vi "Main.vi"() -> ()   [LabVIEW 2015]
doc: "This software acquires data from a simulated source, displays it and performs analysis of the data."
uses:
  Controls/State.ctl
  Controls/Data.ctl
  Controls/Configuration Settings.ctl
  Controls/File Type.ctl
panel:
  in  "File Type":T1
  in  "Open File Location":bool
  in  "Open":bool
  in  "Save":bool
  out "Current State":string
  out "Data":dbl[](graph)
  in  "Reset Settings":bool
  in  "Clear Graph":bool
  in  "Analyze Data":bool
  in  "Acquire Data":bool
  in  "Configure Data":bool
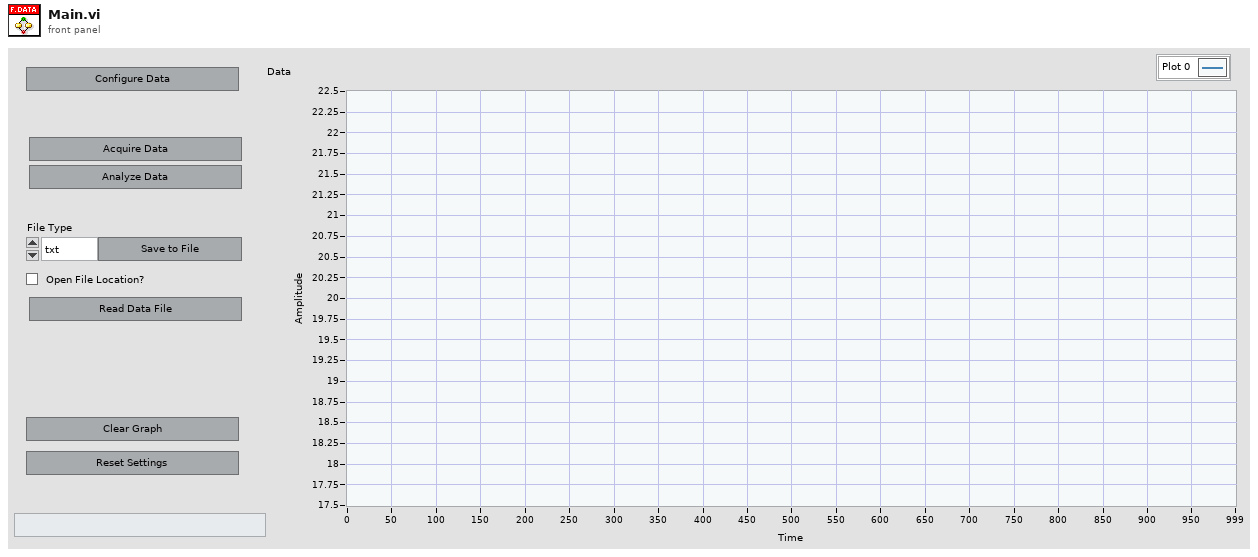
[diagram p1: front panel]
types:
  T1 = typedef "File Type.ctl" = enum16{"txt", "csv", "tdms"}
  T2 = typedef "Data.ctl" = cluster{"Configuration Settings":T3, "Data":dbl[]}
  T3 = typedef "Configuration Settings.ctl" = cluster{"Offset":dbl, "Signal Type":enum16{"Sine Wave", "Triangle Wave", "Square Wave", "Sawtooth Wave"}, "Frequency":dbl, "Amplitude":dbl, "Phase":dbl, "Noise Amplitude":dbl}
  T4 = typedef "State.ctl" = enum16{"Initialize", "Wait for Event", "Configure", "Acquire Data", "Update User Interface", "Reset Data", "Open Data File", "Save Data File", "Clear Data", "Analyse Data", "Stop", "Error"}
  T5 = enum16{"Sine Wave", "Triangle Wave", "Square Wave", "Sawtooth Wave"}
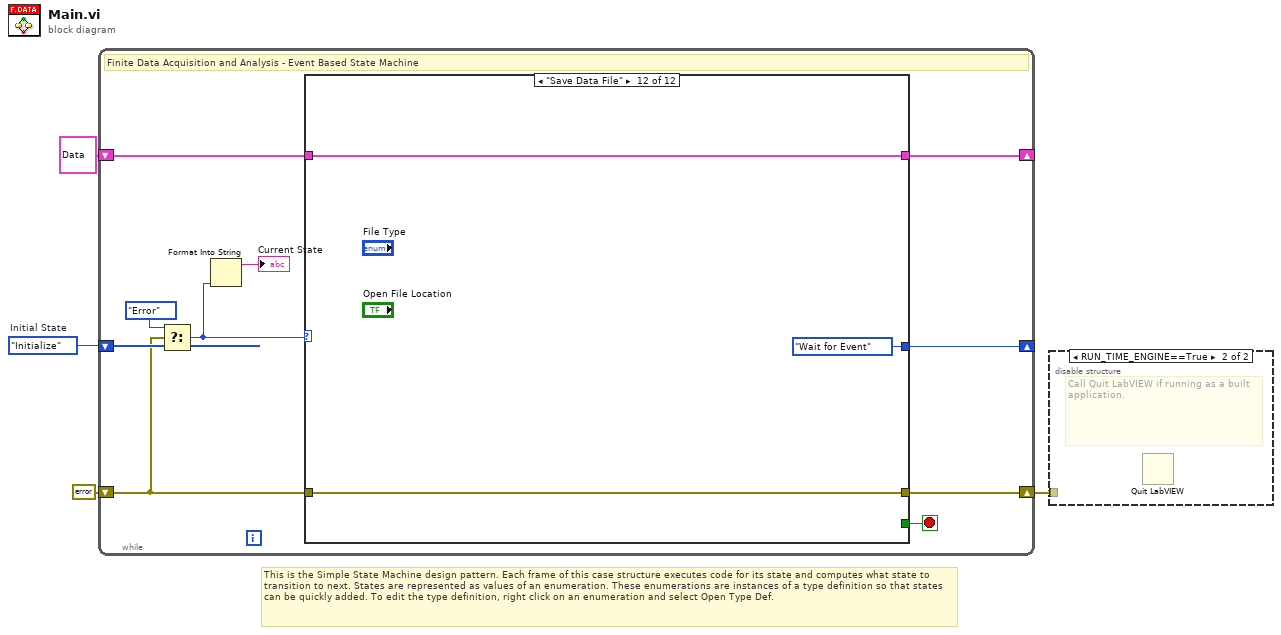
[diagram p0: block diagram]
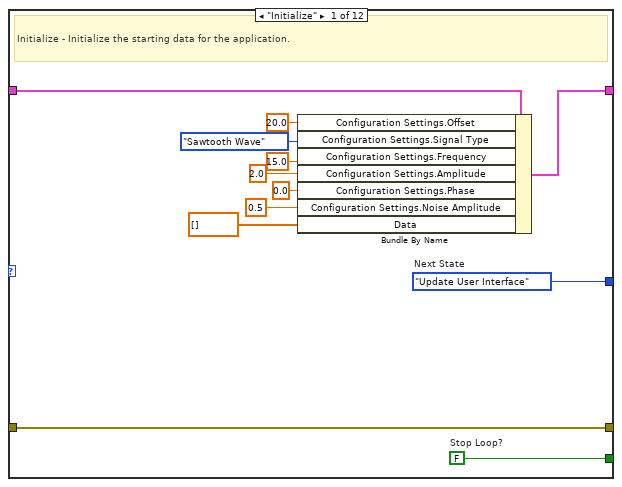
[diagram p2: hidden frame]
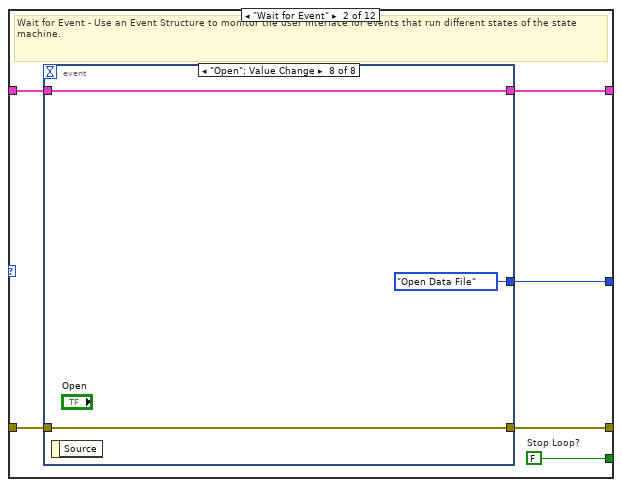
[diagram p3: hidden frame]
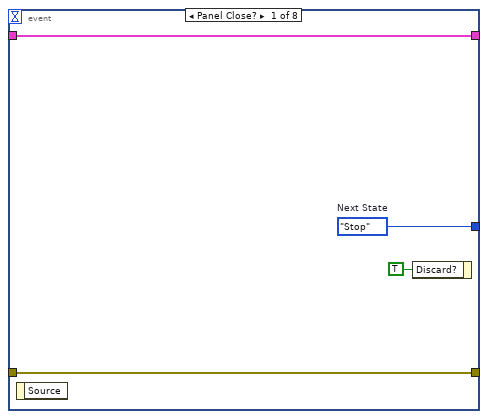
[diagram p4: hidden frame]
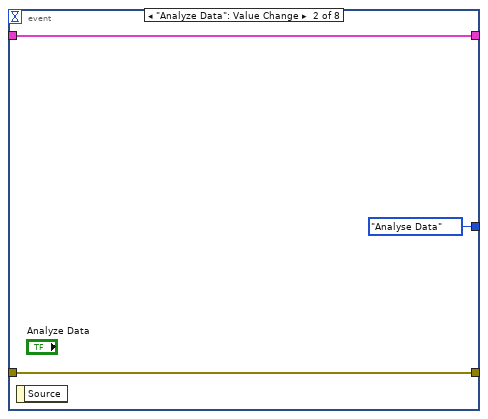
[diagram p5: hidden frame]
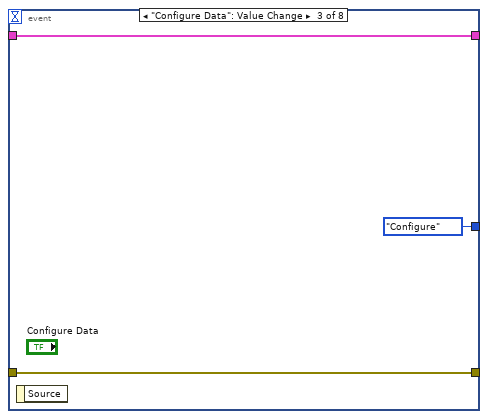
[diagram p6: hidden frame]
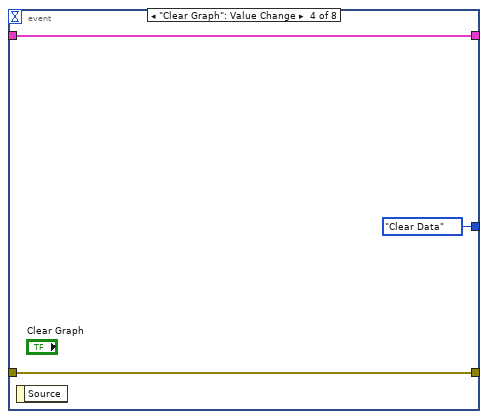
[diagram p7: hidden frame]
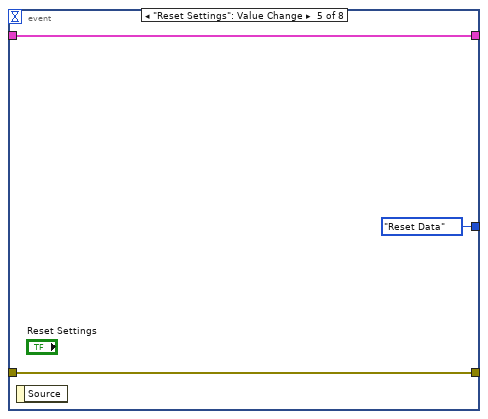
[diagram p8: hidden frame]
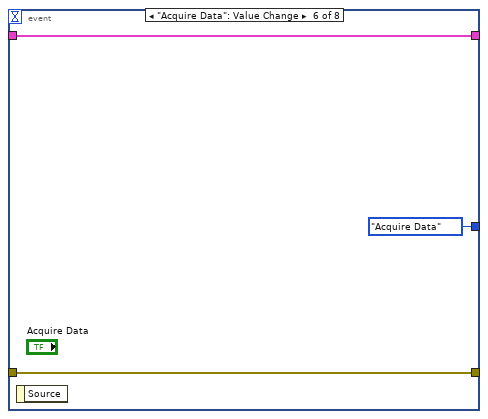
[diagram p9: hidden frame]
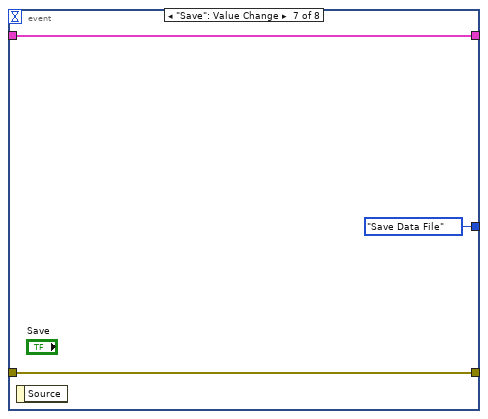
[diagram p10: hidden frame]
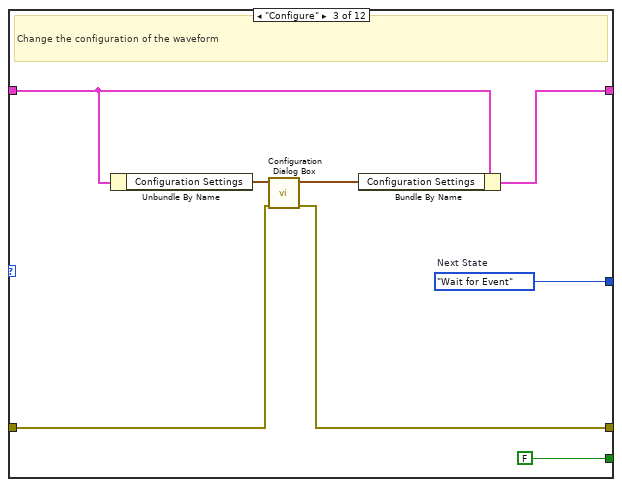
[diagram p11: hidden frame]
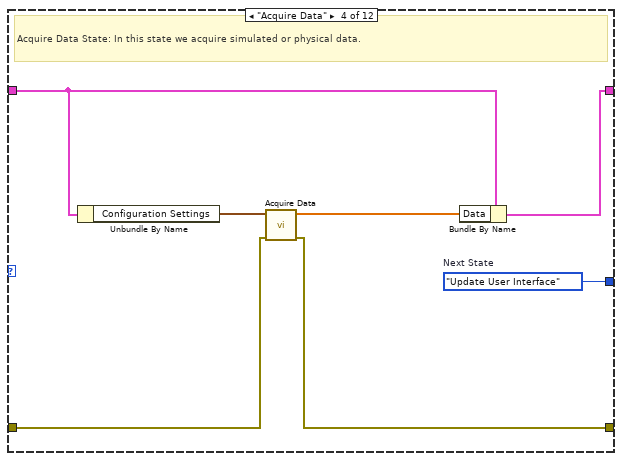
[diagram p12: hidden frame]
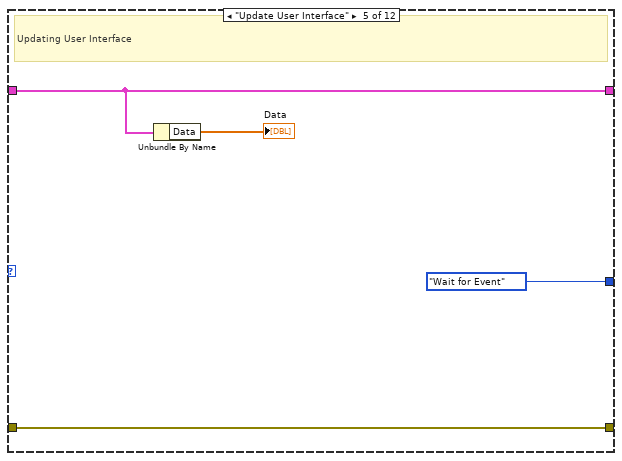
[diagram p13: hidden frame]
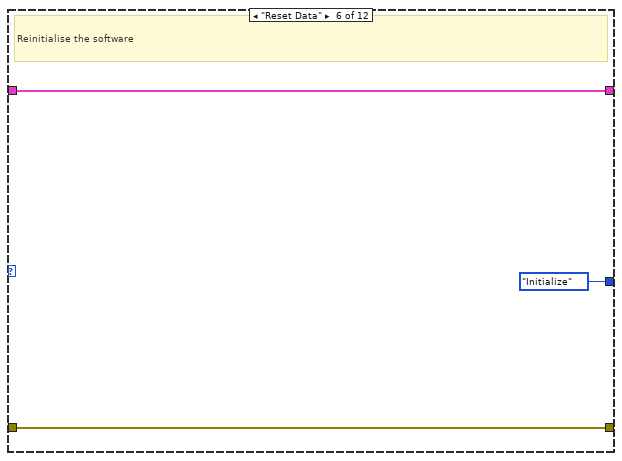
[diagram p14: hidden frame]
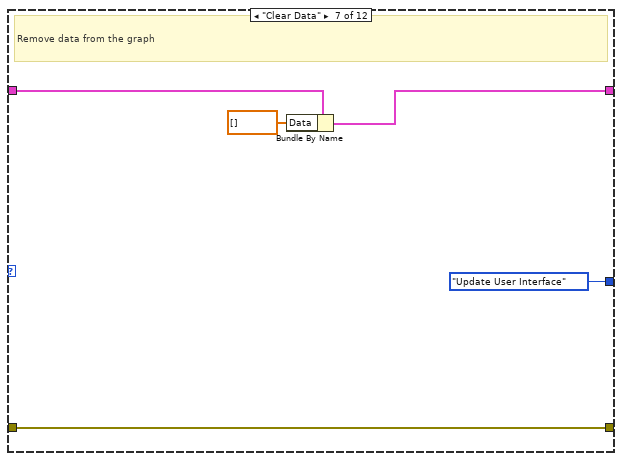
[diagram p15: hidden frame]
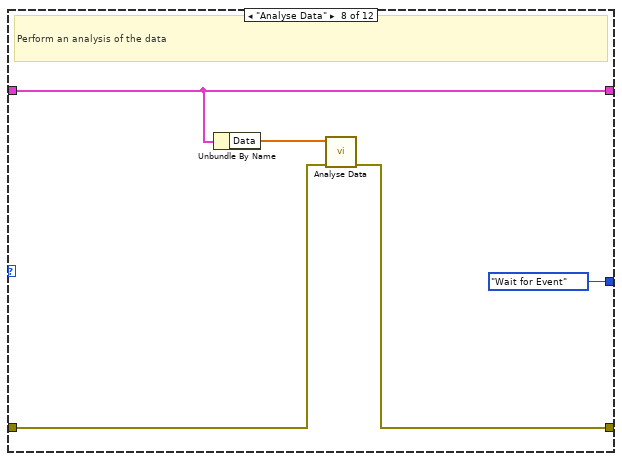
[diagram p16: hidden frame]
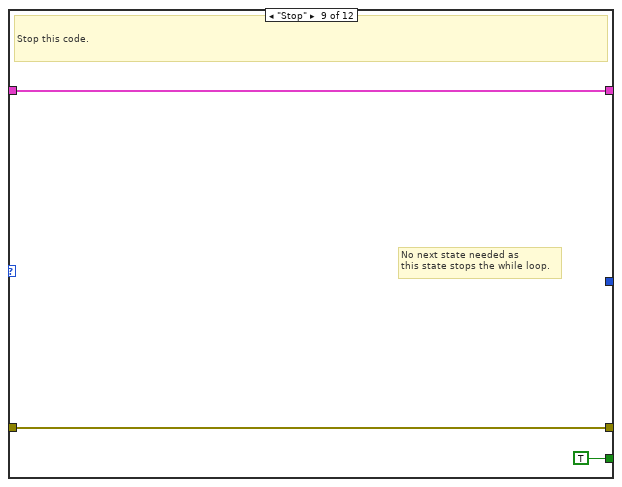
[diagram p17: hidden frame]
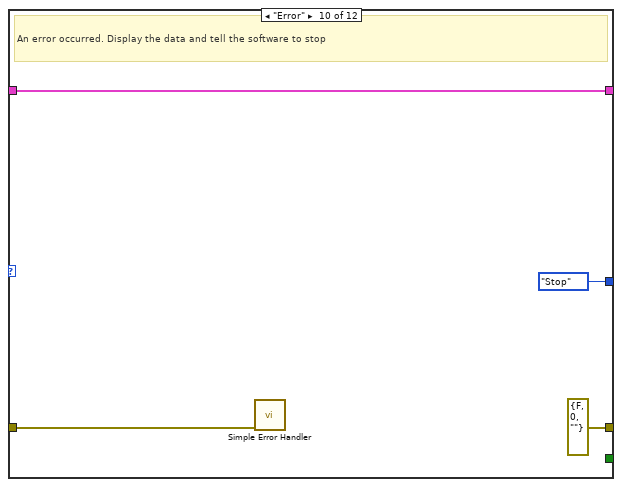
[diagram p18: hidden frame]
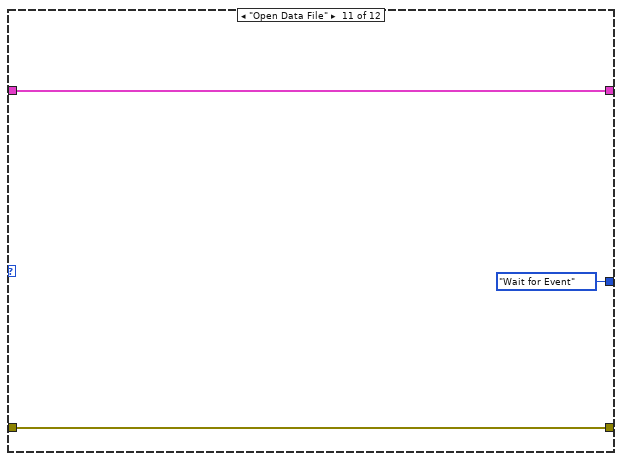
[diagram p19: hidden frame]
diagram:
  w4 = State."Initialize"  # Initial State
  # "This is the Simple State Machine design pattern. Each frame of this case structure executes code for its state and computes what state to transition to next. States are represented as values of an enumeration. These enumerations are instances of a type definition so that states can be quickly added. To edit the type definition, right click on an enumeration and select Open Type Def."
  n1 = while {
    shift-right: [w14] -> _
    shift-left: w4 -> [w9]
    shift-right: [w12] -> _
    shift-left: T2 {"Configuration Settings"={"Offset"=0.0, "Signal Type"=enum."Sine Wave", "Frequency"=10.0, "Amplitude"=1.0, "Phase"=0.0, "Noise Amplitude"=1.0}, "Data"=[]} ("Data") -> [w13]
    shift-right: [w11] -> w1
    shift-left: errorcluster {"status"=FALSE, "code"=0, "source"=""} ("error constant") -> [w10]
    stop <- w5 stop-if-true
    # "Finite Data Acquisition and Analysis - Event Based State Machine"
    n2 = Select(t=State."Error", s=w10, f=w9) -> (s? t:f=w7:T4)
    n3 = Format Into String(w7) -> (resulting string=→"Current State":string)  [unwired: 3 in, 1 out]
    n4 = case shown="\"Save Data File\"" w7 {
      tunnel: [w26 w32 w65 w72 State."Wait for Event" ("(Value Not Used)") State."Initialize" ("(Value Not Used)") State."Update User Interface" ("(Value Not Used)") State."Wait for Event" ("(Value Not Used)") _ State."Stop" ("(Value Not Used)") State."Wait for Event" ("(Value Not Used)") State."Wait for Event" ("(Value Not Used)")] -> w14
      tunnel: [w25 w31 FALSE ("Stop Loop?") _ _ _ _ _ TRUE ("Stop Loop?") _ _ _] -> w5
      tunnel: w13 -> [w24 w30 w60 w68 w74 w79 w84 w86 w92 w96 w99 w102]
      tunnel: [w23 w29 w58 w66 w74 w79 w81 w86 w92 w96 w99 w102] -> w12
      tunnel: w10 -> [w22 w28 w63 w71 w75 w78 w83 w88 w91 w94 w98 w101]
      tunnel: [w22 w27 w62 w70 w75 w78 w83 w87 w91 errorcluster {"status"=FALSE, "code"=0, "source"=""} ("error constant") w98 w101] -> w11
      frame "Initialize" {
        w25 = FALSE  # Stop Loop?
        w26 = State."Update User Interface"  # Next State
        # "Initialize - Initialize the starting data for the application."
        n5 = Bundle By Name(cluster=w24, "Configuration Settings.Offset"=20.0, "Configuration Settings.Signal Type"=T5."Sawtooth Wave", "Configuration Settings.Frequency"=15.0, "Configuration Settings.Amplitude"=2.0, "Configuration Settings.Phase"=0.0, "Configuration Settings.Noise Amplitude"=0.5, "Data"=dbl[] []) -> (w23:T2)
      }
      frame "Wait for Event" {
        w31 = FALSE  # Stop Loop?
        # "Wait for Event - Use an Event Structure to monitor the user interface for events that run different states of the state machine."
        n6 = event shown="[7] \"Open\": Value Change" {
          selector: _ -> [_ _ _ _ _ _ _ _]
          dyn-events: _ -> [_ _ _ _ _ _ _ _]
          timeout: _ -> [_ _ _ _ _ _ _ _]
          tunnel: [w36 State."Analyse Data" ("Next State") State."Configure" ("Next State") State."Clear Data" ("Next State") State."Reset Data" ("Next State") State."Acquire Data" ("Next State") State."Save Data File" ("Next State") State."Open Data File" ("Next State")] -> w32
          tunnel: w30 -> [w35 w39 w42 w45 w48 w51 w54 w57]
          tunnel: [w35 w39 w42 w45 w48 w51 w54 w57] -> w29
          tunnel: w28 -> [w34 w38 w41 w44 w47 w50 w53 w56]
          tunnel: [w34 w38 w41 w44 w47 w50 w53 w56] -> w27
          event Panel Close? {
            w36 = State."Stop"  # Next State
            n7 = event-data() -> ()  [unwired: 1 in, 1 out]
            n8 = event-data("Discard?"=TRUE) -> ()  [unwired: 1 in, 1 out]
          }
          event "Analyze Data": Value Change {
            n9 = event-data() -> ()  [unwired: 1 in, 1 out]
          }
          event "Configure Data": Value Change {
            n10 = event-data() -> ()  [unwired: 1 in, 1 out]
          }
          event "Clear Graph": Value Change {
            n11 = event-data() -> ()  [unwired: 1 in, 1 out]
          }
          event "Reset Settings": Value Change {
            n12 = event-data() -> ()  [unwired: 1 in, 1 out]
          }
          event "Acquire Data": Value Change {
            n13 = event-data() -> ()  [unwired: 1 in, 1 out]
          }
          event "Save": Value Change {
            n14 = event-data() -> ()  [unwired: 1 in, 1 out]
          }
          event "Open": Value Change {
            n15 = event-data() -> ()  [unwired: 1 in, 1 out]
          }
        }
      }
      frame "Configure" {
        w65 = State."Wait for Event"  # Next State
        # "Change the configuration of the waveform"
        n16 = Unbundle By Name(w60) -> ("Configuration Settings"=w61:T3)
        n17 = call "Configuration Dialog Box.vi"("error in (no error)"=w63, "Configuration Settings In"=w61) -> ("error out"=w62:errorcluster, "Configuration Settings Out"=w59:T3)  [unwired: 8 in]
        n18 = Bundle By Name(cluster=w60, "Configuration Settings"=w59) -> (w58:T2)
      }
      frame "Acquire Data" {
        w72 = State."Update User Interface"  # Next State
        # "Acquire Data State: In this state we acquire simulated or physical data."
        n19 = Unbundle By Name(w68) -> ("Configuration Settings"=w69:T3)
        n20 = call "Acquire Data.vi"("error in (no error)"=w71, "Configuration Settings"=w69) -> ("error out"=w70:errorcluster, "Data Out"=w67:dbl[])  [unwired: 8 in]
        n21 = Bundle By Name(cluster=w68, "Data"=w67) -> (w66:T2)
      }
      frame "Update User Interface" {
        # "Updating User Interface"
        n22 = Unbundle By Name(w74) -> ("Data"=→"Data":dbl[])
      }
      frame "Reset Data" {
        # "Reinitialise the software"
      }
      frame "Clear Data" {
        # "Remove data from the graph"
        n23 = Bundle By Name(cluster=w84, "Data"=dbl[] []) -> (w81:T2)
      }
      frame "Analyse Data" {
        # "Perform an analysis of the data"
        n24 = Unbundle By Name(w86) -> ("Data"=w85:dbl[])
        n25 = call "Analyse Data.vi"("error in (no error)"=w88, "Data In"=w85) -> ("error out"=w87:errorcluster)  [unwired: 9 in]
      }
      frame "Stop" {
        # "No next state needed as \nthis state stops the while loop."
        # "Stop this code."
      }
      frame "Error" {
        # "An error occurred. Display the data and tell the software to stop"
        n26 = call <vilib>:"Simple Error Handler.vi"("error in (no error)"=w94) -> ()  [unwired: 4 in, 5 out]
      }
      frame "Open Data File" {
      }
      frame "Save Data File" {
      }
    }
  }
  n27 = disable-structure shown="RUN_TIME_ENGINE==True" {
    disable-tunnel: w1 -> [_ _]
    frame condition #0 (active) {
    }
    frame condition #1 {
      # "Call Quit LabVIEW if running as a built application."
      n28 = Quit LabVIEW() -> ()  [unwired: 1 in]
    }
  }
